vi "clientstreaming_client.vi"() -> ()   [LabVIEW 2019]
uses:
  Generated_client/RPC Messages/Request.ctl
  Generated_client/RPC Messages/Request_request_oneof/Request_request_oneof.lvclass
  Generated_client/RPC Messages/Request_request_oneof/Request_request_oneof.lvclass/Request_request_oneof.ctl
  Generated_client/RPC Messages/Response_response_oneof/Response_response_oneof.lvclass/Response_response_oneof.ctl
  Generated_client/Generated_client.lvlib
  Generated_client/RPC Messages/Response_response_oneof/Response_response_oneof.lvclass
  examples/route_guide/route_guide_client/route_guide_client.lvlib
panel:
  out "error out":errorcluster
  out "result":string
  out "resp_id":i32
  out "new_age":i32
  in  "num_requests":i32
  in  "error in":errorcluster
  in  "age":i32
  in  "req_id":i32
  in  "message":string
  in  "req_oneof":enum16{"message", "req_id"}(ring)
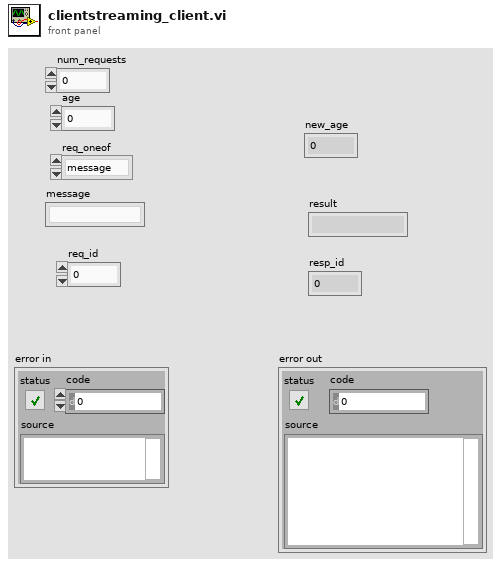
[diagram p1: front panel]
types:
  T1 = typedef "grpc-lvsupport-release.lvlib/grpcId.ctl" = u64
  T2 = typedef "Generated_client.lvlib/Request.ctl" = cluster{"age":i32, "Request_request_oneof":refnum<class "Request_request_oneof.lvclass">}
  T3 = typedef "Generated_client.lvlib/Response.ctl" = cluster{"new_age":i32, "Response_response_oneof":refnum<class "Response_response_oneof.lvclass">}
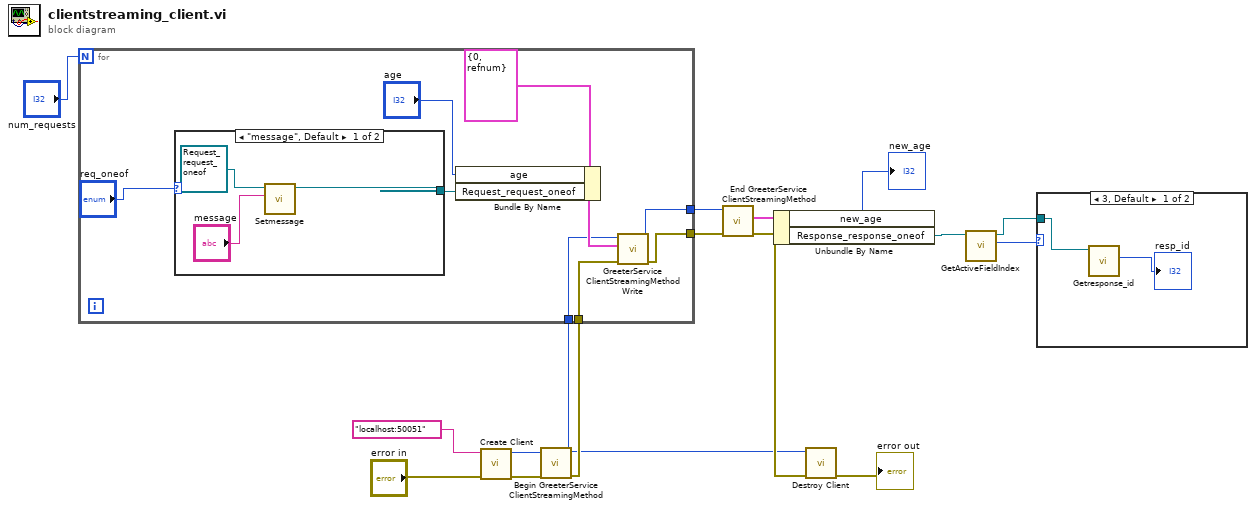
[diagram p0: block diagram]
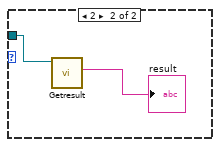
[diagram p2: hidden frame]
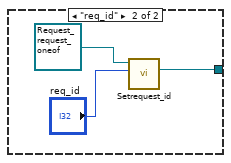
[diagram p3: hidden frame]
diagram:
  n1 = call "Create Client.vi"("error in"="error in", "address"="localhost:50051") -> ("error out"=w15:errorcluster, "gRPC ID Out"=w5:T1)  [unwired: 8 in]
  n2 = call "Begin GreeterService ClientStreamingMethod.vi"("error in"=w15, "gRPC ID"=w5) -> ("error out"=w13:errorcluster, "Call Id Out"=w1:T1, "gRPC ID out"=w2:T1)  [unwired: 7 in]
  n3 = for {
    N: "num_requests" -> [_]
    tunnel: w13 -> [w22]
    tunnel: w1 -> [w20]
    tunnel: [w19] -> w12
    tunnel: [w18] -> w11
    n4 = case shown="\"message\", Default" "req_oneof" {
      tunnel: [w27 w30] -> w25
      frame "message", Default {
        n5 = call "Setmessage.vi"("Set_Val"="message", "OneOfTemplate in"=refnum<class "Request_request_oneof.lvclass"> refnum) -> ("OneOfTemplate out"=w27:refnum<class "Request_request_oneof.lvclass">)  [unwired: 8 in, 1 out]
      }
      frame "req_id" {
        n6 = call "Setrequest_id.vi"("Set_Val"="req_id", "OneOfTemplate in"=refnum<class "Request_request_oneof.lvclass"> refnum) -> ("OneOfTemplate out"=w30:refnum<class "Request_request_oneof.lvclass">)  [unwired: 8 in, 1 out]
      }
    }
    n7 = Bundle By Name(cluster=T2 {"age"=0, "Request_request_oneof"=refnum} ("Request"), "age"="age", "Request_request_oneof"=w25) -> (w21:T2)
    n8 = call "GreeterService ClientStreamingMethod Write.vi"("error in"=w22, "Request Data"=w21, "Call ID in"=w20) -> ("error out"=w19:errorcluster, "Call ID"=w18:T1)  [unwired: 6 in, 1 out]
  }
  n9 = call "End GreeterService ClientStreamingMethod.vi"("error in"=w12, "Call ID in"=w11) -> ("error out"=w4:errorcluster, "Response Data"=w10:T3)  [unwired: 7 in, 1 out]
  n10 = Unbundle By Name(w10) -> ("new_age"=→"new_age":i32, "Response_response_oneof"=w8:refnum<class "Response_response_oneof.lvclass">)
  n11 = call "Destroy Client.vi"("error in"=w4, "gRPC ID"=w2) -> ("error out"=→"error out":errorcluster)  [unwired: 9 in]
  n12 = call "GetActiveFieldIndex.vi"("OneOfTemplate in"=w8) -> ("Active Field Index"=w7:i32, "OneOfTemplate out"=w6:refnum<class "Response_response_oneof.lvclass">)  [unwired: 8 in, 1 out]
  n13 = case shown="3, Default" w7 {
    tunnel: w6 -> [w33 w35]
    frame 3, Default {
      n14 = call "Getresponse_id.vi"("OneOfTemplate in"=w33) -> ("Get_Val"=→"resp_id":i32)  [unwired: 8 in, 2 out]
    }
    frame 2 {
      n15 = call "Getresult.vi"("OneOfTemplate in"=w35) -> ("Get_Val"=→"result":string)  [unwired: 8 in, 2 out]
    }
  }
